vi "ROOT - Release Session.vi"(0 "OBJ - Session in":refnum<class "Session - Root.lvclass">, 5 "Session Handle in":T1, 11 "error in (no error)":errorcluster, 13 "force destroy? (F)":bool) -> (4 "OBJ - Session out":refnum<class "Session - Root.lvclass">, 15 "error out":errorcluster)   [LabVIEW 2018, in "Session - Root.lvclass"]
doc: "Initializes a measurement session\n\nSession data is set to the default values from \"set Defaults.vi\""
uses:
  <userlib>/_Session Fwk/Session - Root.lvclass
  <userlib>/_Session Fwk/Typedefs/Session Handle.ctl
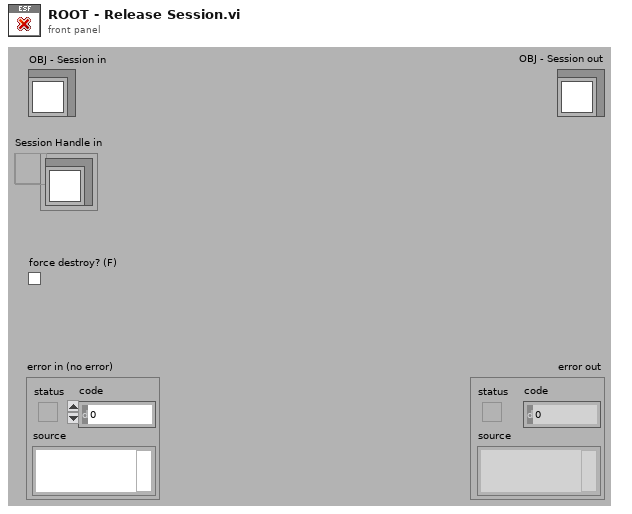
[diagram p1: front panel]
types:
  T1 = typedef "Session - Root.lvclass/Session Handle.ctl" = refnum<data-value>
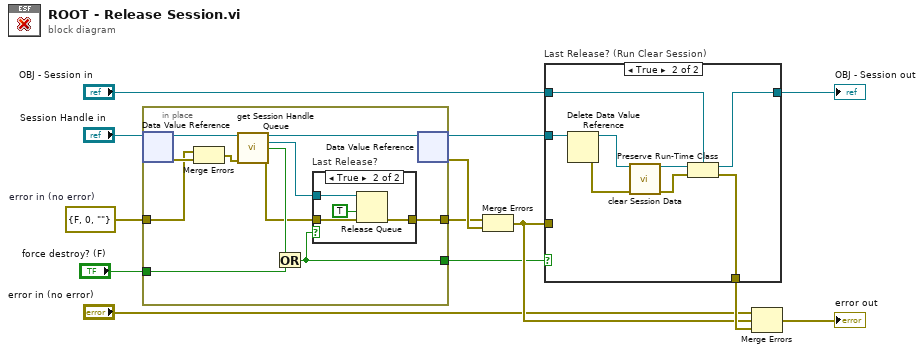
[diagram p0: block diagram]
diagram:
  w3 = errorcluster {"status"=FALSE, "code"=0, "source"=""}  # error in (no error)
  n1 = in-place {
    in-place-border: [w14] -> w1
    in-place-border: "force destroy? (F)" -> [w16]
    in-place-border: w3 -> [w19]
    in-place-border: [w17] -> w2
    n2 = in-place-dvr #1("Session Handle in") -> (w24:refnum<class "Session - Root.lvclass">, w21:errorcluster)
    n3 = Merge Errors(w19, w21) -> (w20:errorcluster)
    n4 = call <userlib>:"get Session Handle Queue.vi"("OBJ - Session in"=w24, "error in (no error)"=w20) -> ("OBJ - Session out"=w23:refnum<class "Session - Root.lvclass">, "Session Queue Handle"=w18:refnum<queue>, "Last Session?"=w22:bool, "error out"=w15:errorcluster)  [unwired: 10 in]
    n5 = Or(x=w22, y=w16) -> (x .or. y?=w14:bool)
    n6 = case "Last Release?" shown="True" w14 {
      tunnel: w18 -> [_ w29]
      tunnel: [w25 w28] -> w17
      tunnel: w15 -> [w25 w27]
      frame False {
      }
      frame True {
        n7 = Release Queue(queue=w29, force destroy? (F)=TRUE, error in (no error)=w27) -> (error out=w28:errorcluster)  [unwired: 2 out]
      }
    }
    n8 = in-place-dvr #1(w23) -> (w9:T1, w8:errorcluster)
  }
  n9 = Merge Errors(w2, w8) -> (w5:errorcluster)
  n10 = case "Last Release? (Run Clear Session)" shown="True" w1 {
    tunnel: "OBJ - Session in" -> [w31 w37]
    tunnel: [w31 w34] -> w12
    tunnel: w9 -> [_ w39]
    tunnel: w5 -> [w30 _]
    tunnel: [w30 w32] -> w7
    frame False {
    }
    frame True {
      n11 = Delete Data Value Reference(data value reference=w39) -> (data value=w38:refnum<class "Session - Root.lvclass">, error out=w33:errorcluster)  [unwired: 1 in]
      n12 = call-dynamic "clear Session Data.vi"("OBJ - Measurement Session in"=w38, "error in"=w33) -> ("OBJ - Measurement Session out"=w35:refnum<class "Session - Root.lvclass">, "error out"=w36:errorcluster)  [unwired: 12 in]
      n13 = Preserve Run-Time Class(object in=w35, error in=w36, 2:w37) -> (object out=w34:refnum<class "Session - Root.lvclass">, error out=w32:errorcluster)
    }
  }
  "OBJ - Session out" <- w12
  n14 = Merge Errors("error in (no error)", w5, w7) -> (→"error out":errorcluster)
